vi "DHE_DRV_get_cont_read.vi"(8 "error in (no error)":errorcluster, 11 "fd":i32) -> (0 "error out":errorcluster, 2 "cont_read":i32, 3 "fd":i32)   [LabVIEW 2016]
doc: "This VI closes the I/O interface with the instrument."
uses:
  c/lib/libarcDHE.so
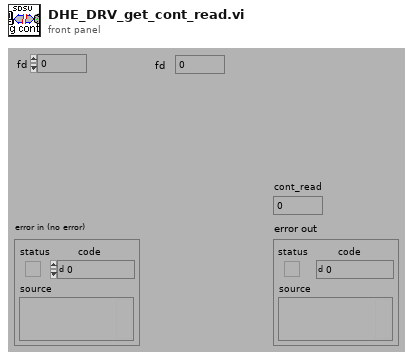
[diagram p1: front panel]
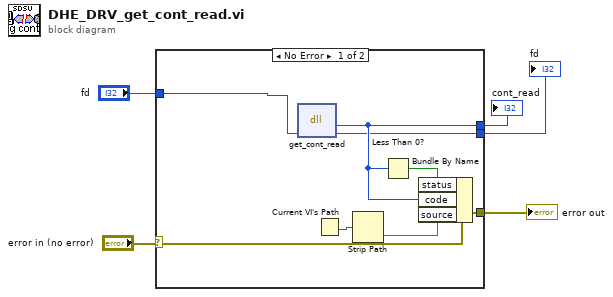
[diagram p0: block diagram]
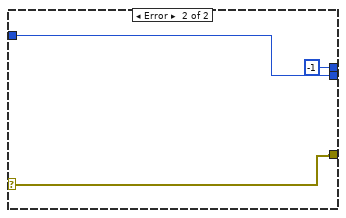
[diagram p2: hidden frame]
diagram:
  n1 = case shown="No Error" "error in (no error)" {
    selector: "error in (no error)" -> [w7 w16]
    tunnel: [w12 -1] -> w5
    tunnel: [w9 w16] -> w4
    tunnel: [w8 w15] -> w3
    tunnel: "fd" -> [w6 w15]
    frame No Error {
      n2 = dll-call lib="home/simager/panview/PAN/Modules/SDSU/private/c/lib/libarcDHE.so" fn="get_cont_read" label="cont_read"("fd"=w6) -> (w12:i32, "fd"=w8:i32)  [unwired: 3 in, 2 out]
      n3 = Current VI's Path() -> (path=w11:path)
      n4 = Strip Path(path=w11) -> (name=w10:string)  [unwired: 1 out]
      n5 = Less Than 0?(x=w12) -> (x < 0?=w13:bool)
      n6 = Bundle By Name(cluster=w7, "status"=w13, "code"=w12, "source"=w10) -> (w9:errorcluster)
    }
    frame Error {
    }
  }
  "error out" <- w4
  "cont_read" <- w5
  "fd" <- w3
